vi "Create Interface.vi"(7 "App Inst":refnum<vi>, 8 "error in (no error)":errorcluster, 9 "Actor Name":string, 11 "Library in":refnum<vi>) -> (0 "error out":errorcluster, 3 "Library out":refnum<vi>)   [LabVIEW 2020, in "Add Actor Interface.lvlib"]
uses:
  Add Actor Interface.lvlib
  <vilib>/Utility/EditLVLibs/Edit LVLibs.lvlib
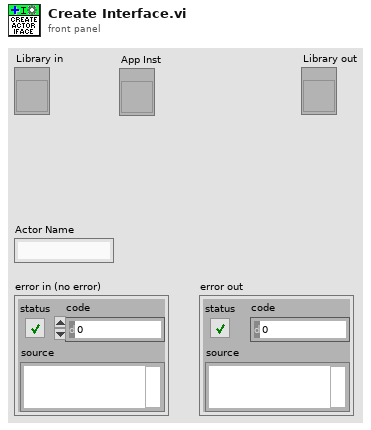
[diagram p1: front panel]
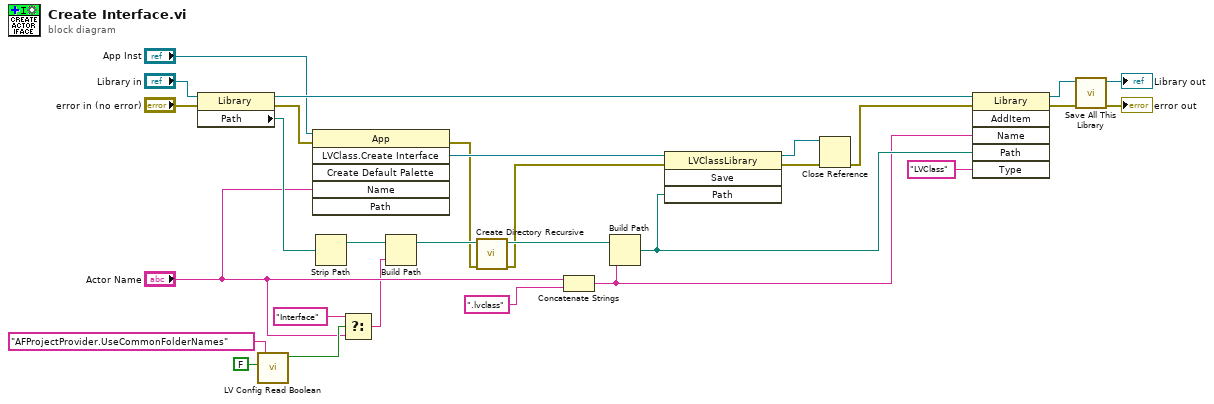
[diagram p0: block diagram]
diagram:
  n1 = property class="Library"(reference="Library in", error in="error in (no error)") -> (reference out=w28:refnum<vi>, error out=w22:errorcluster, "Path"=w26:path)
  n2 = call <resource>:"LV Config Read Boolean.vi"("default value"=FALSE, "key"="AFProjectProvider.UseCommonFolderNames") -> ("value"=w4:bool)  [unwired: 3 in, 2 out]
  n3 = invoke class="App" method="LVClass.Create Interface"(reference="App Inst", error in=w22, "Name"="Actor Name") -> (error out=w13:errorcluster, "LVClass.Create Interface"=w21:refnum<vi>)  [unwired: 3 in, 4 out]
  n4 = Strip Path(path=w26) -> (stripped path=w17:path)  [unwired: 1 out]
  n5 = Select(t="Interface", s=w4, f="Actor Name") -> (s? t:f=w1:string)
  n6 = Build Path(base path=w17, name or relative path=w1) -> (appended path=w15:path)
  n7 = call <vilib>:"Create Directory Recursive.vi"("error in (no error)"=w13, "directory"=w15) -> ("error out"=w12:errorcluster, "directory copy"=w14:path)  [unwired: 3 in, 1 out]
  n8 = Concatenate Strings("Actor Name", ".lvclass" ("string")) -> (w16:string)
  n9 = Build Path(base path=w14, name or relative path=w16) -> (appended path=w24:path)
  n10 = invoke class="LVClassLibrary" method="Save"(reference=w21, error in=w12, "Path"=w24) -> (reference out=w20:refnum<vi>, error out=w19:errorcluster)  [unwired: 1 in, 2 out]
  n11 = Close Reference(reference=w20, error in (no error)=w19) -> (error out=w18:errorcluster)
  n12 = invoke class="Library" method="AddItem"(reference=w28, error in=w18, "Name"=w16, "Path"=w24, "Type"="LVClass") -> (reference out=w8:refnum<vi>, error out=w10:errorcluster)  [unwired: 1 in, 4 out]
  n13 = call <vilib>:"Save All This Library.vi"("error in (no error)"=w10, "Library in"=w8) -> ("error out"=→"error out":errorcluster, "Library out"=→"Library out":refnum<vi>)  [unwired: 8 in]
